vi "Local_Path_New_Stop(SubVI).vi"(0 "x_lat_arr":dbl[](array[numeric]), 2 "WP no_pre":i32, 5 "y_long_arr":dbl[](array[numeric]), 7 "vel_arr":dbl[](array[numeric]), 9 "x_lat_c":dbl, 11 "y_long_c":dbl, 12 "evt_arr":dbl[](array[numeric]), 13 "# of pnt":i32) -> (4 "INDEX(Near Point)":i32, 6 "Evt(Local)":dbl[](array[numeric]), 8 "Lat(Local)":dbl[](array[numeric]), 10 "Long(Local)":dbl[](array[numeric]), 15 "Vel(Local)":dbl[](array[numeric]))   [LabVIEW 2024]
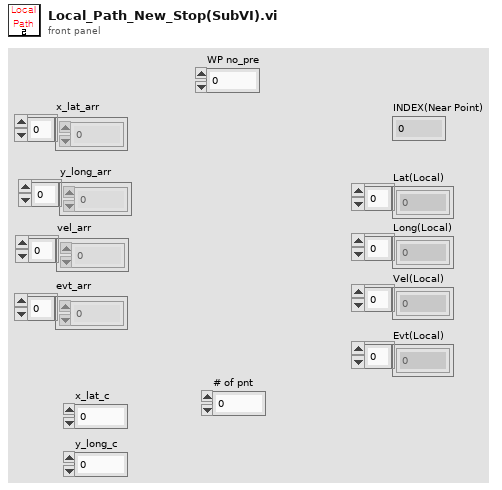
[diagram p1: front panel]
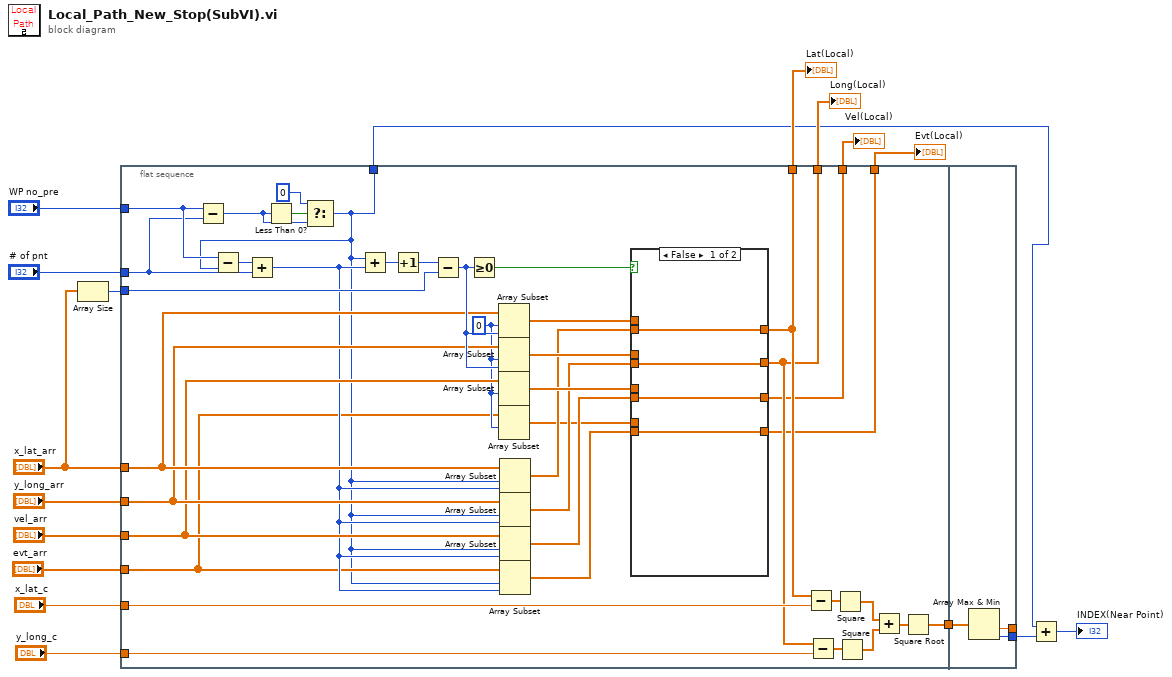
[diagram p0: block diagram]
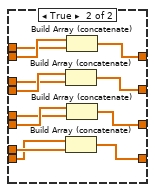
[diagram p2: hidden frame]
diagram:
  n1 = Array Size(array="x_lat_arr") -> (size(s)=w7:i32)
  n2 = flat-sequence {
    tunnel: "WP no_pre" -> [w51]
    tunnel: "# of pnt" -> [w50]
    tunnel: "x_lat_arr" -> [w37]
    tunnel: "y_long_arr" -> [w36]
    tunnel: "x_lat_c" -> [w44]
    tunnel: "y_long_c" -> [w43]
    tunnel: [w42] -> w12
    tunnel: "vel_arr" -> [w35]
    tunnel: w7 -> [w39]
    tunnel: [w27] -> w6
    tunnel: [w26] -> w5
    tunnel: [w25] -> w4
    tunnel: "evt_arr" -> [w21]
    tunnel: [w19] -> w2
    tunnel: [w18] -> w1
    tunnel: w12 -> [w74]
    tunnel: [w73] -> _
    tunnel: [w72] -> w11
    frame #0 {
      w22 = 0 ("인덱스")
      n3 = Subtract(x=w51, y=w50) -> (x-y=w54:i32)
      n4 = Less Than 0?(x=w54) -> (x < 0?=w55:bool)
      n5 = Select(t=0, s=w55, f=w54) -> (s? t:f=w18:i32)
      n6 = Subtract(x=w51, y=w18) -> (x-y=w53:i32)
      n7 = Add(x=w53, y=w50) -> (x+y=w24:i32)
      n8 = Add(x=w18, y=w24) -> (x+y=w41:i32)
      n9 = Increment(x=w41) -> (x+1=w40:i32)
      n10 = Subtract(x=w40, y=w39) -> (x-y=w38:i32)
      n11 = Greater Or Equal To 0?(x=w38) -> (x >= 0?=w34:bool)
      n12 = Array Subset(array=w37, index=w22, length=w38) -> (w33:dbl[])
      n13 = Array Subset(array=w36, index=w22, length=w38) -> (w32:dbl[])
      n14 = Array Subset(array=w35, index=w22) -> (w31:dbl[])  [unwired: 1 in]
      n15 = Array Subset(array=w21, index=w22) -> (w20:dbl[])  [unwired: 1 in]
      n16 = Array Subset(array=w37, index=w18, length=w24) -> (w28:dbl[])
      n17 = Array Subset(array=w36, index=w18, length=w24) -> (w29:dbl[])
      n18 = Array Subset(array=w35, index=w18, length=w24) -> (w30:dbl[])
      n19 = Array Subset(array=w21, index=w18, length=w24) -> (w23:dbl[])
      n20 = case shown="False" w34 {
        tunnel: w28 -> [w59 w71]
        tunnel: w33 -> [_ w70]
        tunnel: w32 -> [_ w63]
        tunnel: w29 -> [w58 w64]
        tunnel: [w59 w69] -> w27
        tunnel: [w58 w68] -> w26
        tunnel: w30 -> [w57 w67]
        tunnel: w31 -> [_ w66]
        tunnel: [w57 w65] -> w25
        tunnel: w23 -> [w56 w61]
        tunnel: w20 -> [_ w62]
        tunnel: [w56 w60] -> w19
        frame False {
        }
        frame True {
          n21 = Build Array (concatenate)(w64, w63) -> (w68:dbl[])
          n22 = Build Array (concatenate)(w61, w62) -> (w60:dbl[])
          n23 = Build Array (concatenate)(w71, w70) -> (w69:dbl[])
          n24 = Build Array (concatenate)(w67, w66) -> (w65:dbl[])
        }
      }
      n25 = Subtract(x=w27, y=w44) -> (x-y=w49:dbl[])
      n26 = Subtract(x=w26, y=w43) -> (x-y=w48:dbl[])
      n27 = Square(x=w49) -> (x^2=w47:dbl[])
      n28 = Square(x=w48) -> (x^2=w46:dbl[])
      n29 = Add(x=w47, y=w46) -> (x+y=w45:dbl[])
      n30 = Square Root(x=w45) -> (sqrt(x)=w42:dbl[])
    }
    frame #1 {
      n31 = Array Max & Min(array=w74) -> (min value=w73:dbl, min index (indices)=w72:i32)  [unwired: 2 out]
    }
  }
  n32 = Add(x=w1, y=w11) -> (x+y=→"INDEX(Near Point)":i32)
  "Lat(Local)" <- w6
  "Long(Local)" <- w5
  "Vel(Local)" <- w4
  "Evt(Local)" <- w2
